vi "SLSC Convert EDS Property to VS Channel.vi"(0 "Section Ptr":T1 format="%.0x", 1 "GUID Get Properties Page":string, 2 "GUID Set Properties Page":string, 3 "Documentation":string, 5 "property":T2, 7 "Physical Channel":string, 9 "SLSCChannelPath":string, 11 "error in (no error)":errorcluster, 12 "enums":T3[](array[typedef])) -> (4 "Parent Ref out":T1 format="%.0x", 15 "error out":errorcluster)   [LabVIEW 2020, in "SLSC CD System Explorer.lvlib"]
uses:
  SLSC CD System Explorer.lvlib
  SLSC EDS API/JSON parsing/enum.ctl
  <vilib>/NI VeriStand/Custom Device API/Custom Device Item Ref.ctl
  SLSC EDS API/JSON parsing/property.ctl
  <vilib>/NI VeriStand/Custom Device API/Custom Device API.lvlib
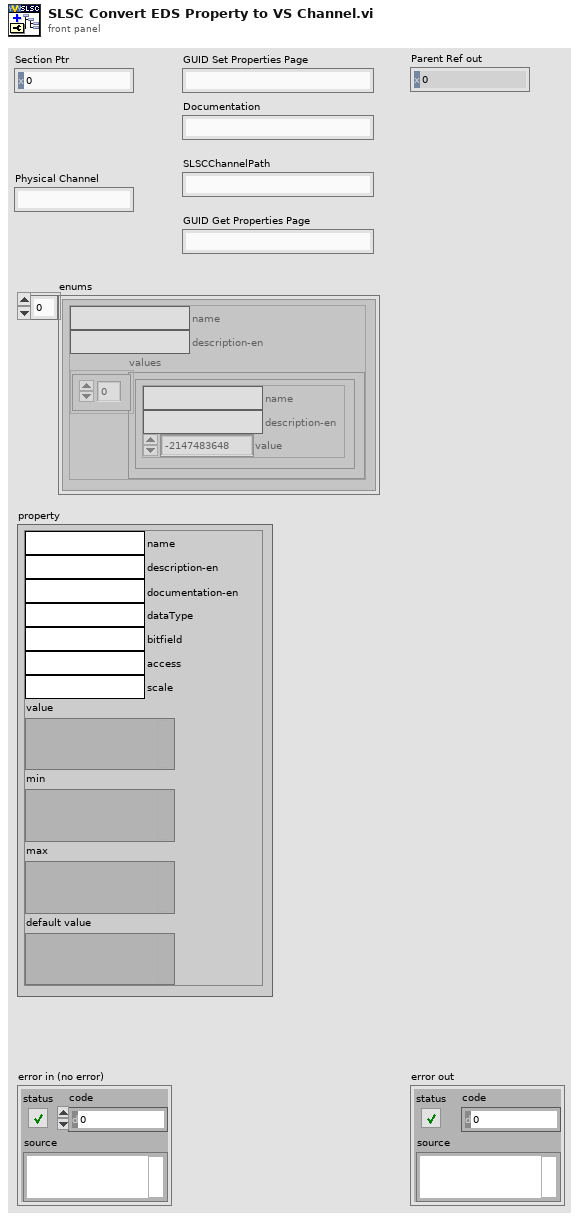
[diagram p1: front panel]
types:
  T1 = typedef "Custom Device API.lvlib/Custom Device Item Ref.ctl" = u64
  T2 = typedef "property.ctl" = cluster{"name":string, "description-en":string, "documentation-en":string, "dataType":string, "bitfield":string, "access":string, "scale":string, "value":variant, "min":variant, "max":variant, "default value":variant}
  T3 = typedef "enum.ctl" = cluster{"name":string, "description-en":string, "values":cluster{"name":string, "description-en":string, "value":i32}[]}
  T4 = typedef "Custom Device API.lvlib/Custom Device Channel.ctl" = cluster{"Type":T5, "Units":string, "Default Value":dbl, "Faultable":bool, "Scalable":bool}
  T5 = typedef "Custom Device API.lvlib/Custom Device Channel Type.ctl" = enum16{"Input", "Output"}
  T6 = cluster{"Name":string, "Enum Names":string[], "Enum Values":i32[]}
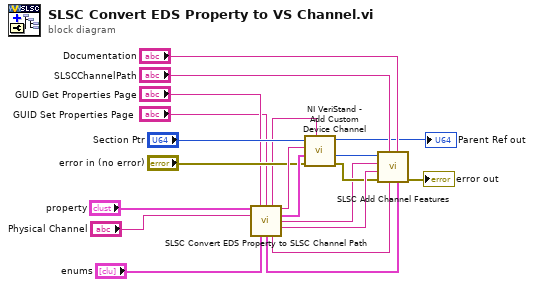
[diagram p0: block diagram]
diagram:
  n1 = call "SLSC Convert EDS Property to SLSC Channel Path.vi"("property"="property", "GUID Get Properties Page"="GUID Get Properties Page", "GUID Set Properties Page"="GUID Set Properties Page", "Physical Channel"="Physical Channel", "enums"="enums") -> ("GUID Properties Page"=w2:string, "name"=w8:string, "Channel out"=w9:T4, "SLSC Channel Path"=w14:string, "documentation-en"=w16:string, "Cluster"=w1:T6, "description-en"=w17:string)  [unwired: 4 in]
  n2 = call <vilib>:"NI VeriStand - Add Custom Device Channel.vi"("GUID (Default Channel)"=w2, "error in (no error)"="error in (no error)", "Channel"=w9, "Channel Name"=w8, "Parent Ref in"="Section Ptr") -> ("error out"=w15:errorcluster, "Channel Ref"=w13:T1, "Parent Ref out"=→"Parent Ref out":T1)  [unwired: 3 in, 1 out]
  n3 = call "SLSC Add Channel Features.vi"("Cluster Enum"=w1, "Documentation"="Documentation", "description-en"=w17, "SLSCChannelPath"="SLSCChannelPath", "error in (no error)"=w15, "documentation-en"=w16, "SLSC Command Name"=w14, "Channel Ref"=w13) -> ("error out"=→"error out":errorcluster)  [unwired: 2 in, 1 out]
